vi "Get Events.vi"(11 "Create Test Node View in":refnum<class "Create Test Node View.lvclass">) -> (2 "Events":T1, 3 "Create Test Node View out":refnum<class "Create Test Node View.lvclass">)   [LabVIEW 2013, in "Create Test Node View.lvlib" / "Create Test Node View.lvclass"]
uses:
  Create Test Node View.lvclass
  Typedef/Events.ctl
  Create Test Node View.lvclass/Create Test Node View.ctl
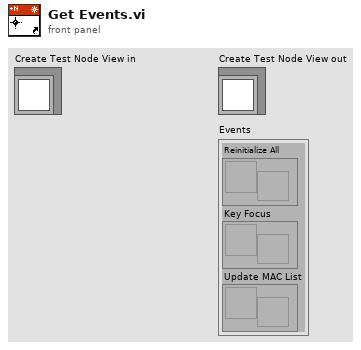
[diagram p1: front panel]
types:
  T1 = typedef "Create Test Node View.lvlib/Create Test Node View.lvclass/Events.ctl" = cluster{"Reinitialize All":refnum<user-event>, "Key Focus":refnum<user-event>, "Update MAC List":refnum<user-event>}
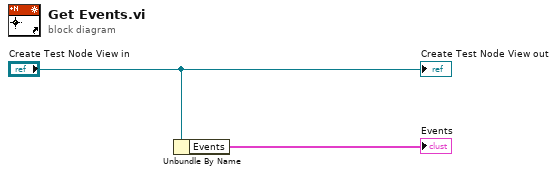
[diagram p0: block diagram]
diagram:
  n1 = Unbundle By Name("Create Test Node View in") -> ("Events"=→"Events":T1)
  "Create Test Node View out" <- "Create Test Node View in"
